vi "Generate Random Obstacles.vi"(8 "obstacle cost":dbl, 9 "free cost":dbl, 10 "chance":dbl, 11 "cost in":dbl[][](array[numeric])) -> (3 "cost out":dbl[][](array[numeric]))   [LabVIEW 2012]
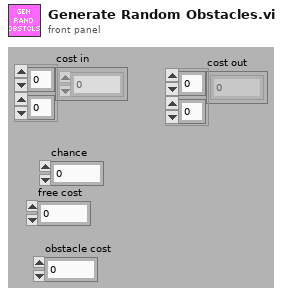
[diagram p1: front panel]
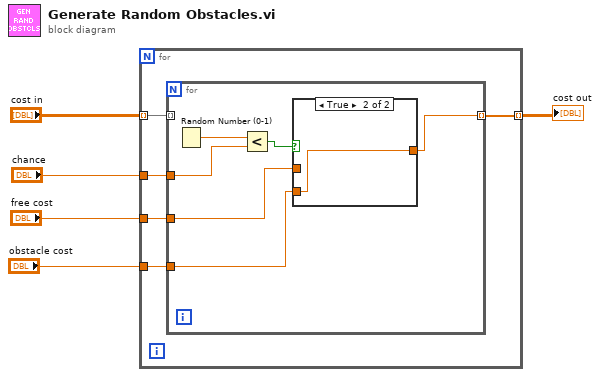
[diagram p0: block diagram]
diagram:
  n1 = for {
    tunnel: "cost in" -> [w10] mode=indexing
    tunnel: [w9] -> w4 mode=indexing
    tunnel: "chance" -> [w8]
    tunnel: "obstacle cost" -> [w7]
    tunnel: "free cost" -> [w6]
    n2 = for {
      tunnel: w10 -> [_] mode=indexing
      tunnel: [w11] -> w9 mode=indexing
      tunnel: w8 -> [w15]
      tunnel: w7 -> [w13]
      tunnel: w6 -> [w12]
      n3 = Random Number (0-1)() -> (number: 0 to 1=w16:dbl)
      n4 = Less?(x=w16, y=w15) -> (x < y?=w14:bool)
      n5 = case shown="True" w14 {
        tunnel: w13 -> [_ w18]
        tunnel: w12 -> [w17 _]
        tunnel: [w17 w18] -> w11
        frame False {
        }
        frame True {
        }
      }
    }
  }
  "cost out" <- w4
